vi "tatrocki_target_C1.vi"   [LabVIEW 2020]
uses:
  <vilib>/Platform/TimedLoop/XDataNode/timing_clust.ctl
  <vilib>/Platform/TimedLoop/XDataNode/nitl_modes.ctl
  <vilib>/Platform/TimedLoop/XDataNode/wakeup.ctl
  <vilib>/platform/TimedLoop/XDataNode/XDataNode.xnode
  <vilib>/Platform/TimedLoop/XDataNode/XDNodeRunTimeDep.lvlib
types:
  T1 = typedef "XDNodeRunTimeDep.lvlib/timing_clust.ctl" = cluster{"Expected End [f-1]":u64, "Actual End [f-1]":u64, "Finished Late? [f-1]":bool, "Expected End [i-1]":u64, "Actual End [i-1]":u64, "Finished Late? [i-1]":bool, "Expected Start [i]":u64, "Actual Start [i]":u64, "Expected Start [f]":u64, "Actual Start [f]":u64, "Source Name":string, "Structure Name":string, "Period":i64, "Deadline":i64, "Offset":i64, "Start":i64, "Priority":i32, "Timeout":i32, "Mode":T2, "Wakeup Reason":T3, "Error":errorcluster, "Source Type":string, "Secondary Source Type":string, "Global End Time":u64, "Global Start Time":u64, "Frame Duration":u64, "Iteration Duration":u64, "Assigned CPU":i32, "I/O Scan Engine Mode":u32}
  T2 = typedef "XDNodeRunTimeDep.lvlib/nitl_modes.ctl" = enum32{"No Change", "Process missed periods, maintain original phase", "Discard missed periods, maintain original phase", "Process missed periods, ignore original phase", "Discard missed periods, ignore original phase"}
  T3 = typedef "XDNodeRunTimeDep.lvlib/wakeup.ctl" = enum32{"Normal", "Aborted", "Asynchronous wakeup", "Timing source error", "Timed loop error", "Timeout"}
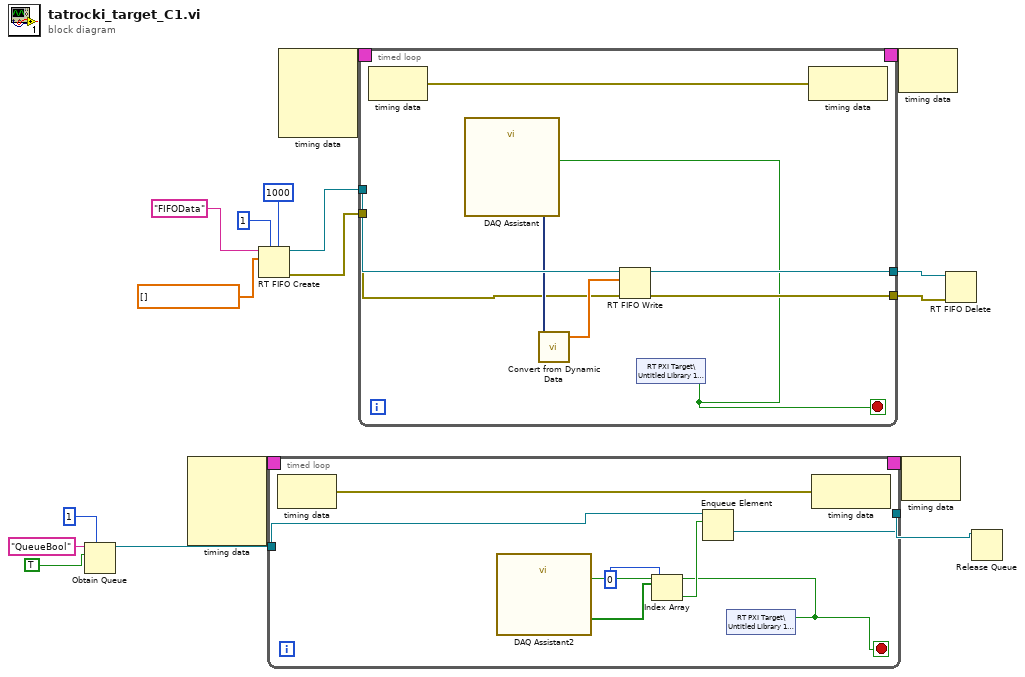
[diagram p0: block diagram]
diagram:
  n1 = Obtain Queue(max queue size (-1, unlimited)=1, name (unnamed)="QueueBool", element data type=TRUE) -> (queue out=w2:refnum<queue>)  [unwired: 2 in, 2 out]
  n2 = node-c288() -> (w7:T1)  [unwired: 4 in]
  n3 = RT FIFO Create(0:"FIFOData" ("name (unnamed)"), 1:dbl[] [], 4:u32 1 ("size (10)"), 6:u32 1000 ("elements in array (1)")) -> (8:w11:refnum<k33>, 11:w10:errorcluster)  [unwired: 4 in, 1 out]
  n4 = timed-loop {
    timing: w7 -> [_]
    timing-out: [_] -> w6
    tunnel: w2 -> [w23]
    tunnel: [w22] -> w1
    stop <- w18 stop-if-true
    n5 = node-c288() -> (w24:errorcluster)  [unwired: 1 in]
    n6 = shared-variable "RT PXI Target\\Untitled Library 1.lvlib\\Stop"() -> (w18:bool)  [unwired: 1 in, 1 out]
    n7 = call "DAQ Assistant2"("stop (T)"=w18) -> ("data"=w21:bool[])  [unwired: 16 in, 2 out]
    n8 = Index Array(array=w21, index=0) -> (element=w19:bool)
    n9 = Enqueue Element(queue=w23, element=w19) -> (queue out=w22:refnum<queue>)  [unwired: 2 in, 2 out]
    n10 = node-c288(w24) -> ()  [unwired: 1 out]
  }
  n11 = node-c288() -> (w17:T1)  [unwired: 4 in]
  n12 = timed-loop {
    timing: w17 -> [_]
    timing-out: [_] -> w16
    tunnel: w11 -> [w36]
    tunnel: w10 -> [w33]
    tunnel: [w32] -> w9
    tunnel: [w31] -> w8
    stop <- w30 stop-if-true
    n13 = node-c288() -> (w37:errorcluster)  [unwired: 1 in]
    n14 = shared-variable "RT PXI Target\\Untitled Library 1.lvlib\\Stop"() -> (w30:bool)  [unwired: 1 in, 1 out]
    n15 = call "DAQ Assistant"("stop (T)"=w30) -> ("data"=w35:dynamicdata)  [unwired: 16 in, 2 out]
    n16 = call "Convert from Dynamic Data"("Dynamic Data Type"=w35) -> ("Array"=w34:dbl[])  [unwired: 3 in]
    n17 = RT FIFO Write(0:w36, 1:w34, 3:w33) -> (8:w32:refnum<k33>, 11:w31:errorcluster)  [unwired: 2 in, 2 out]
    n18 = node-c288(w37) -> ()  [unwired: 1 out]
  }
  n19 = node-c288(w16) -> ()  [unwired: 1 out]
  n20 = node-c288(w6) -> ()  [unwired: 1 out]
  n21 = RT FIFO Delete(0:w9, 3:w8) -> ()  [unwired: 1 in, 1 out]
  n22 = Release Queue(queue=w1) -> ()  [unwired: 2 in, 3 out]
